vi "whilw structure 2.vi"() -> ()   [LabVIEW 2020]
panel:
  in  "Boolean":bool
  out "Respuesta":i32
  in  "Numeric 2":i32
  out "Numeric":i32
  in  "Stop buttom":bool
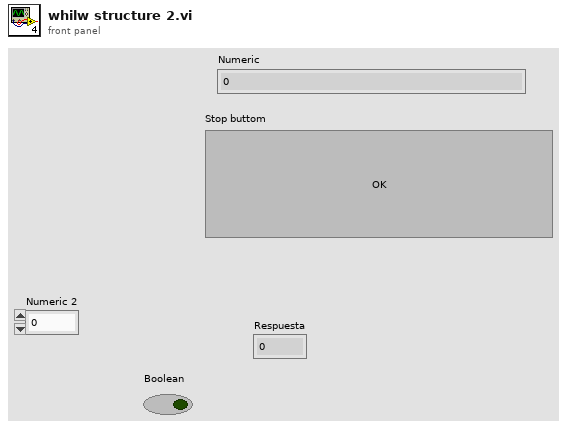
[diagram p1: front panel]
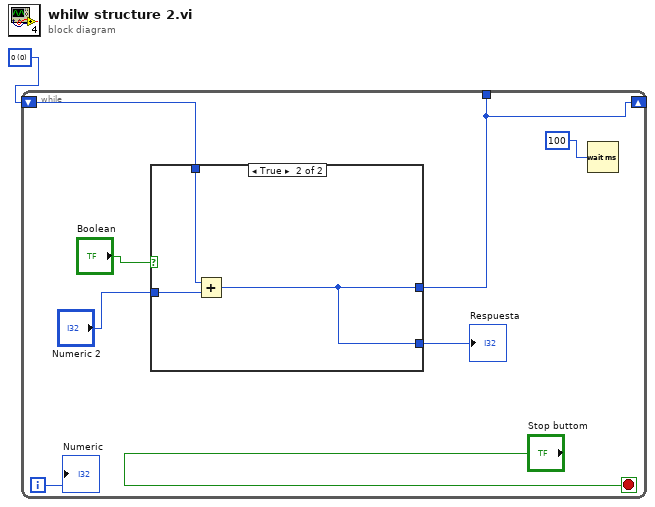
[diagram p0: block diagram]
diagram:
  w1 = u16 0 items=["0"]
  n1 = while {
    tunnel: [w3] -> _
    shift-right: [w3] -> _
    shift-left: w1 -> [w4]
    i -> [w7]
    stop <- "Stop buttom" stop-if-true
    n2 = case shown="True" "Boolean" {
      tunnel: "Numeric 2" -> [_ w12]
      tunnel: w4 -> [w9 w11]
      tunnel: [w9 w10] -> w3
      tunnel: [w9 w10] -> _
      frame False {
      }
      frame True {
        n3 = Add(x=w11, y=w12) -> (x+y=w10:i32)
      }
    }
    "Respuesta" <- w3
    n4 = Wait (ms)(milliseconds to wait=u32 100 ("millisecond timer value")) -> ()  [unwired: 1 out]
    "Numeric" <- w7
  }
